vi "TestRunner_Init.vi"(8 "error in (no error)":errorcluster, 10 "publicEvents":T1, 11 "TextTestRunner in":refnum<class "TestRunner.lvclass">) -> (0 "error out":errorcluster, 3 "TextTestRunner out":refnum<class "TestRunner.lvclass">)   [LabVIEW 2013, in "TestRunner.lvclass"]
uses:
  TestRunner.lvclass
  PublicEvents--Cluster.ctl
  TestResult/resultStatusChanged--Cluster.ctl
  TestResult/resultStatus--enum.ctl
  TestResult/testStarted--Cluster.ctl
  TestRunner.lvclass/TestRunner.ctl
  TestResult/TestResult.lvclass
panel:
  # "JKI VI Tester for LabVIEW\nhttp://jkisoft.com/vi-tester\nCopyright (C) 2007-2009, JKI <info@jkisoft.com>\nALL RIGHTS RESERVED"
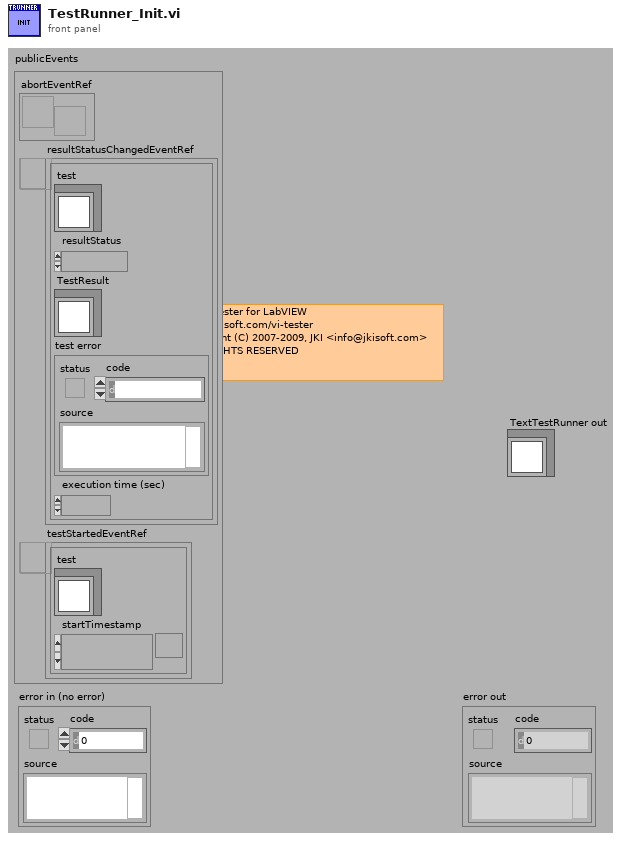
[diagram p1: front panel]
types:
  T1 = typedef "TestRunner.lvclass/PublicEvents--Cluster.ctl" = cluster{"abortEventRef":refnum<user-event>, "resultStatusChangedEventRef":refnum<user-event>, "testStartedEventRef":refnum<user-event>}
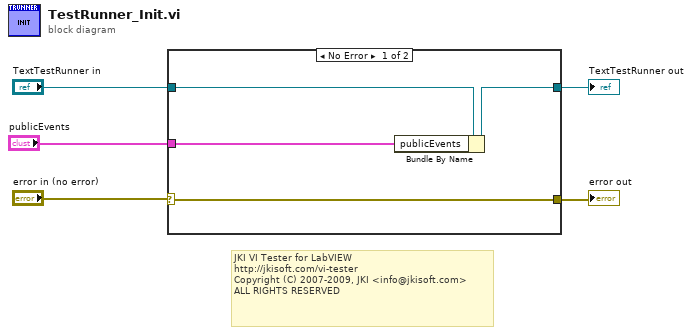
[diagram p0: block diagram]
diagram:
  # "JKI VI Tester for LabVIEW\nhttp://jkisoft.com/vi-tester\nCopyright (C) 2007-2009, JKI <info@jkisoft.com>\nALL RIGHTS RESERVED"
  n1 = case shown="No Error" "error in (no error)" {
    selector: "error in (no error)" -> [w7 w10]
    tunnel: "TextTestRunner in" -> [w9 w11]
    tunnel: [w8 w11] -> w4
    tunnel: [w7 w10] -> w2
    tunnel: "publicEvents" -> [w6 _]
    frame No Error {
      n2 = Bundle By Name(cluster=w9, "publicEvents"=w6) -> (w8:refnum<class "TestRunner.lvclass">)
    }
    frame Error {
    }
  }
  "TextTestRunner out" <- w4
  "error out" <- w2
